vi "Main.vi"(10 "Parameters":variant, 11 "Process":refnum<class "Process.lvclass">) -> ()   [LabVIEW 2015, in "J1939 Addon Engine.lvlib"]
uses:
  J1939 Addon Engine.lvlib
  <vilib>/NI/NI VeriStand Inline Async API/_VS Inline Async API/Process/Process.lvclass
  Types/Process Parameters.ctl
  Shared/Types/XNET Settings.ctl
  Types/Incoming Single Point Configuration.ctl
  Types/Incoming Single Point Frame Pairs.ctl
  Shared/Types/Incoming Single Point Channel Pairs.ctl
  <vilib>/NI Veristand/Custom Device API/Data Reference.ctl
  Types/Outgoing Cyclic Configuration.ctl
  Types/Outgoing Cyclic Frame Pairs.ctl
  Shared/Types/XNET Frame Event Properties.ctl
  Shared/Types/Outgoing Cyclic Channel Pairs.ctl
  <vilib>/NI Veristand/Custom Device API/Block Data Reference.ctl
  Shared/Types/Monitor Settings.ctl
  Types/Simulated Settings.ctl
  Shared/Types/Compiled Simulated Settings.ctl
  Types/DTC FIFOs.ctl
  <vilib>/NI/NI VeriStand Inline Async API/_VS Inline Async API/Process/Process.lvclass/Process.ctl
  Shared/J1939 Multi Packet Frame/SubVIs/Convert Frame to NI-XNET CAN Frame.vi
  Shared/J1939 Multi Packet Frame/SubVIs/Listen for Claim.vi
  Shared/J1939 Multi Packet Frame/SubVIs/Address Claim Address.vi
  Shared/J1939 Utilities/Common Conversions.vi
  Shared/J1939 Utilities/SubVIs/Convert CAN Data (U8) to U32.vi
  Network Address Lookup Table.vi
  Shared/J1939 Multi Packet Frame/SubVIs/Cannont Claim Address.vi
  Shared/J1939 Utilities/SubVIs/Convert CAN Data (U32) to U8.vi
  Convert Signals to Frame by ID.vi
  Data Lookup Table Set Signals (Range).vi
  Data Lookup Table Get Signals (Range).vi
  <vilib>/NI/NI VeriStand Inline Async API/_VS Inline Async API/Process/Methods/Async.Processes.Report.vi
  Shared/J1939 Multi Packet Frame/Process Outgoing Messages.vi
  Shared/J1939 Multi Packet Frame/Check Outgoing TP Timeouts.vi
  Shared/J1939 Multi Packet Frame/SubVIs/Read Queued Processed Outgoing Messages.vi
  Shared/J1939 Multi Packet Frame/SubVIs/Read Queued Processed Incoming Messages.vi
  Conversion Lookup Table Get Conversion Parameter.vi
  Shared/J1939 Multi Packet Frame/SubVIs/RQST Look for Response.vi
  Shared/J1939 Multi Packet Frame/Check Incoming TP Timeouts.vi
  Shared/J1939 Multi Packet Frame/Process Incoming Messages.vi
  Shared/J1939 Multi Packet Frame/SubVIs/RQST Comm Lookup Table_Actions.vi
  Shared/J1939 Multi Packet Frame/SubVIs/RQST Wait on Response.vi
  Shared/J1939 Multi Packet Frame/SubVIs/RQST Wait on Multiple Requests.vi
  TCP Check Connection.vi
  Shared/STM/STM Get Connection Reference.vi
  Shared/STM/TCP/STM Get Connection Reference (TCP).vi
  <vilib>/Utility/error.llb/Clear Errors.vi
  Shared/J1939 Utilities/SubVIs/Convert CAN Arb ID to J1939 ID.vi
  Shared/J1939 Utilities/SubVIs/Convert J1939 ID to CAN Arb ID.vi
  <vilib>/NI/NI VeriStand Inline Async API/_VS Inline Async API/Error Handling Process/SubVIs/Error.ConvertArray.vi
  Shared/J1939 Multi Packet Frame/SubVIs/Read Queued Outgoing Messages.vi
  Shared/J1939 Multi Packet Frame/SubVIs/Process Outgoing Messages by Frame Type.vi
  Shared/J1939 Multi Packet Frame/J1939 Periodic Messages/Periodic Message Generator.vi
  Shared/J1939 Multi Packet Frame/SubVIs/Connection Mode Generation Queue Messages.vi
  Shared/J1939 Multi Packet Frame/SubVIs/RQST Lookup Table Act.vi
  Shared/J1939 Multi Packet Frame/J1939 Multi Packet Frames/BAM Buffer.vi
  Shared/J1939 Multi Packet Frame/SubVIs/TP Buffer Check Timeout on Connections.vi
  Shared/J1939 Multi Packet Frame/SubVIs/Buffer Connections List_Actions.vi
  Shared/J1939 Multi Packet Frame/J1939 Multi Packet Frames/Connnection Mode Buffer.vi
  Shared/J1939 Utilities/SubVIs/TP.Conn Abort.vi
  Shared/J1939 Utilities/Filter by Device Address.vi
  Shared/J1939 Multi Packet Frame/SubVIs/Process Incoming Messages by PDU F.vi
  Shared/J1939 Utilities/Common Messages.vi
  Shared/J1939 Utilities/SubVIs/Request.vi
  Shared/J1939 Utilities/Check Output Message Frame Type.vi
  Shared/J1939 Multi Packet Frame/J1939 Multi Packet Frames/BAM Generation.vi
  Shared/J1939 Multi Packet Frame/SubVIs/BAM Generation Connections List_Actions.vi
  Shared/J1939 Multi Packet Frame/SubVIs/BAM Generation Create New TP Connection.vi
  Shared/J1939 Multi Packet Frame/J1939 Multi Packet Frames/Connection Mode Generation.vi
  Shared/J1939 Multi Packet Frame/SubVIs/Connection Mode Generation Connections List_Actions.vi
  Shared/J1939 Multi Packet Frame/SubVIs/Connection Mode Generation Search for Connection (Local Message).vi
  Shared/J1939 Multi Packet Frame/SubVIs/Connection Mode Generation Create New TP Connection.vi
  Shared/J1939 Multi Packet Frame/SubVIs/Connection Mode Generation Get Next Messages.vi
  Shared/J1939 Utilities/Parse Message Type.vi
  Get Simulated Previously Active DTCs.vi
  Get Simulated Active DTCs.vi
  Shared/J1939 Utilities/SubVIs/Acknowledgement.vi
  Shared/J1939 Multi Packet Frame/SubVIs/TP Buffer Search for Connection (No PGN).vi
  Shared/J1939 Multi Packet Frame/SubVIs/TP Buffer Add New Data Packet to Connection.vi
  Shared/J1939 Multi Packet Frame/SubVIs/TP Buffer Convert Connection Info to CAN Frame.vi
  Shared/J1939 Multi Packet Frame/SubVIs/TP Buffer Create New TP Connection.vi
  Shared/J1939 Utilities/SubVIs/TP.CM EndofMsgACK.vi
  Shared/J1939 Utilities/SubVIs/TP.CM CTS.vi
  Shared/J1939 Multi Packet Frame/SubVIs/Connection Mode Generation Search for Connection (Remote Message).vi
  Shared/J1939 Multi Packet Frame/SubVIs/TP Buffer Search for Connection.vi
  Shared/J1939 Multi Packet Frame/SubVIs/Connection Mode Generation CTS Received.vi
  Shared/J1939 Utilities/SubVIs/TP.CM BAM.vi
  Shared/J1939 Utilities/SubVIs/TP.DT.vi
  Shared/J1939 Utilities/SubVIs/TP.CM RTS.vi
  Convert Data to DTC Frame.vi
  Shared/J1939 Utilities/SubVIs/Convert PGN + SA to J1939 ID.vi
  <vilib>/xnet/xnet.llb/XNET Convert.vi
  <vilib>/xnet/xnet.llb/XNET Convert (Signal to Frame Raw).vi
  Data Lookup Table.vi
  Conversion Lookup Table.vi
  Shared/J1939 Multi Packet Frame/SubVIs/Connection Mode Generation Connections List.vi
  Shared/J1939 Multi Packet Frame/SubVIs/BAM Generation Queue Messages.vi
  Shared/J1939 Multi Packet Frame/SubVIs/BAM Generation Connections List.vi
  Shared/J1939 Multi Packet Frame/SubVIs/BAM Generation Search for Connection (Local Message).vi
  <vilib>/xnet/xnet.llb/XNET Write.vi
  <vilib>/xnet/xnet.llb/XNET Write (Frame CAN).vi
  <vilib>/xnet/xnet.llb/XNET Convert (Frame CAN to Signal).vi
  Shared/J1939 Multi Packet Frame/SubVIs/RQST Lookup Table.vi
  Shared/J1939 Multi Packet Frame/SubVIs/BAM Buffer Connections List.vi
  Shared/J1939 Multi Packet Frame/SubVIs/Address Lookup Table.vi
  <vilib>/xnet/xnet.llb/XNET Read.vi
  <vilib>/xnet/xnet.llb/XNET Read (Frame CAN).vi
  Shared/STM/Clear Specific Error.vi
  Shared/STM/Connection Manager/TCP Connection Manager.vi
  <vilib>/NI Veristand/Custom Device Tools/Custom Device Utility Library/NI VeriStand - Print Debug String.vi
  Shared/STM/STM Read Meta Data.vi
  Shared/STM/TCP/STM Read Meta Data (TCP Ref).vi
  Shared/STM/STM Write Message.vi
  Shared/STM/TCP/STM Write Message (TCP).vi
  <vilib>/xnet/xnet.llb/XNET Read (State CAN Comm).vi
  <vilib>/Utility/error.llb/Error Cluster From Error Code.vi
  Shared/STM/STM Read Message.vi
  Shared/STM/TCP/STM Read Message (TCP).vi
  Shared/J1939 Utilities/SubVIs/Request Address.vi
  Shared/J1939 Addon Shared.lvlib
  <vilib>/NI VeriStand/Custom Device API/Custom Device API.lvlib
panel:
  out "error out":errorcluster
  # "CONTROL & MONITORING"
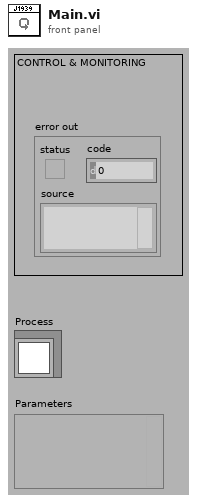
[diagram p1: front panel]
types:
  T1 = typedef "J1939 Addon Engine.lvlib/Process Parameters.ctl" = cluster{"J1939 XNET Settings":T2, "Incoming Single Point Configuraiton":T3, "Outgoing Cyclic Configuraiton":T7, "J1939 Monitor Settings":T12, "Simulated Addresses":T13[], "Simulated Addresses LUT":variant, "Name":string}
  T2 = typedef "J1939 Addon Shared.lvlib/XNET Settings.ctl" = cluster{"XNET Database":refnum<k21>, "XNET Cluster":refnum<k21>, "CAN Port":string, "Baud rate [Bd]":u32, "Termination":u32, "Incoming Rate":u32, "Outcoming Rate":u32, "Write Decimation":u32}
  T3 = typedef "J1939 Addon Engine.lvlib/Incoming Single Point Configuration.ctl" = cluster{"Incoming Single Point Frame":T4, "Channel Pairs":T5, "Read FIFO":refnum<k33>}
  T4 = typedef "J1939 Addon Engine.lvlib/Incoming Single Point Frame Pairs.ctl" = cluster{"ID":u32[], "Conversion":refnum<k21>[], "Channel Array Positions":cluster{"Offset":u32, "Length":u32}[], "Frame Length":u32[]}
  T5 = typedef "J1939 Addon Shared.lvlib/Incoming Single Point Channel Pairs.ctl" = cluster{"Chan Refs":T6[], "Previous Chan Values":dbl[]}
  T6 = typedef "Custom Device API.lvlib/Data Reference.ctl" = i32
  T7 = typedef "J1939 Addon Engine.lvlib/Outgoing Cyclic Configuration.ctl" = cluster{"Outgoing Cyclic Frame":T8, "Channel Pairs":T10, "Write FIFO":refnum<k33>}
  T8 = typedef "J1939 Addon Engine.lvlib/Outgoing Cyclic Frame Pairs.ctl" = cluster{"ID":u32[], "Conversion":refnum<k21>[], "Channel Array Positions":cluster{"Offset":u32, "Length":u32}[], "Frame Length":u32[], "Transmit Propreties":T9[]}
  T9 = typedef "J1939 Addon Shared.lvlib/XNET Frame Event Properties.ctl" = cluster{"Transmit trigger":enum16{"Channel value change"}, "Enable software cyclic trigger":bool, "Transmit Time":dbl}
  T10 = typedef "J1939 Addon Shared.lvlib/Outgoing Cyclic Channel Pairs.ctl" = cluster{"Block Data Refs":T11[], "Previous Chan Values":dbl[]}
  T11 = typedef "Custom Device API.lvlib/Block Data Reference.ctl" = cluster{"Data Reference":T6, "Offset":u64, "Length":u64}
  T12 = typedef "J1939 Addon Shared.lvlib/Monitor Settings.ctl" = cluster{"J1939 Network Address":u8, "Name":u64}
  T13 = typedef "J1939 Addon Engine.lvlib/Simulated Settings.ctl" = cluster{"Simulated Addresses":T14, "FIFOs":T15}
  T14 = typedef "J1939 Addon Shared.lvlib/Compiled Simulated Settings.ctl" = cluster{"J1939 XNET Settings":T12, "DM1 Data":T11[], "DM1 Data":dbl[], "DM1 Enable?":T11[], "DM1 Enable?":dbl[], "DM2 Data":T11[], "DM2 Data":dbl[], "DM2 Enable?":T11[], "DM2 Enable?":dbl[]}
  T15 = typedef "J1939 Addon Engine.lvlib/DTC FIFOs.ctl" = cluster{"DM1 Data":refnum<k33>, "DM1 Enable?":refnum<k33>, "DM2 Data":refnum<k33>, "DM2 Enable?":refnum<k33>, "DM1 Reset?":refnum<k33>, "DM2 Reset?":refnum<k33>}
  T16 = typedef "J1939 Addon Engine.lvlib/Configuration Cluster.ctl" = cluster{"Parameters":T1, "Name":string, "J1939 Cluster":T17, "References":T18, "Frame In":refnum<k21>, "Frame Out":refnum<k21>, "Incoming Timeout":u32, "Outgoing Timeout":u32, "Listener ID":refnum<k5>, "Process":refnum<class "Process.lvclass">, "Data Ref":T24, "Scale Ref":T25, "Incoming Direct Access":cluster{"Offset":u32, "Length":u32}, "Outgoing Direct Access":cluster{"Offset":u32, "Length":u32}, "TCP Mngr Ref":T26, "Name and Address":string, "Simulated Addresses":T13[], "Simulated Addresses LUT":variant}
  T17 = typedef "J1939 Addon Engine.lvlib/Setup Information Cluster.ctl" = cluster{"Processed Incoming":refnum<queue>, "Current Device Address":u8, "Processed Outgoing":refnum<queue>, "Process Outgoing":refnum<queue>, "Name":u64}
  T18 = typedef "J1939 Addon Engine.lvlib/TP List References.ctl" = cluster{"BAM Buffer":T19, "CM Buffer":T19, "CM Gen":T20, "BAM Gen":T21, "Address Claims":T22, "RQST":T23}
  T19 = typedef "J1939 Addon Engine.lvlib/BAM Buffer Connections List_Ref.ctl" = refnum<data-value>
  T20 = typedef "J1939 Addon Engine.lvlib/Connection Mode Generation Connection Ref.ctl" = refnum<data-value>
  T21 = typedef "J1939 Addon Engine.lvlib/BAM Generation Connections List_Ref.ctl" = refnum<data-value>
  T22 = typedef "J1939 Addon Engine.lvlib/Address Table Reference.ctl" = refnum<data-value>
  T23 = typedef "J1939 Addon Engine.lvlib/RQST Lookup Table Reference.ctl" = refnum<data-value>
  T24 = typedef "J1939 Addon Engine.lvlib/Data Lookup Table Reference.ctl" = refnum<data-value>
  T25 = typedef "J1939 Addon Engine.lvlib/Conversion Lookup Table Reference.ctl" = refnum<data-value>
  T26 = typedef "J1939 Addon Shared.lvlib/RQST Comm Lookup Table_Ref.ctl" = refnum<data-value>
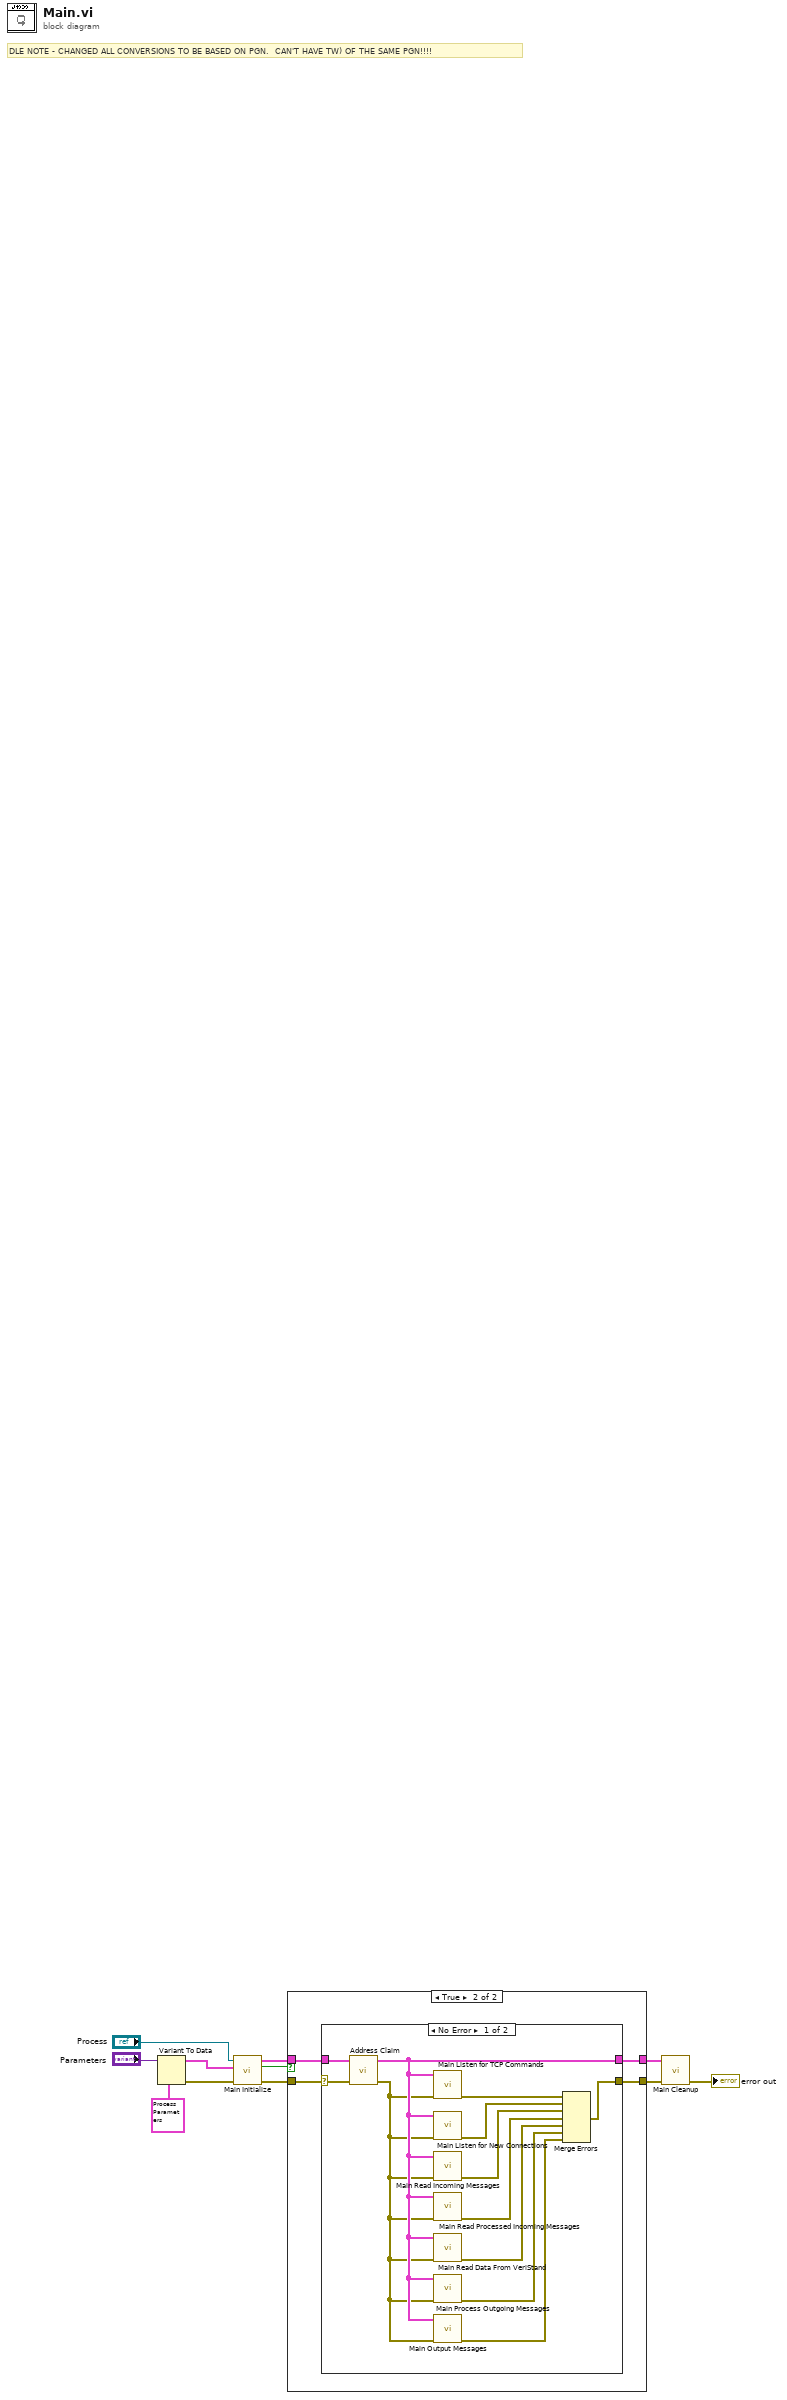
[diagram p0: block diagram]
diagram:
  # "DLE NOTE - CHANGED ALL CONVERSIONS TO BE BASED ON PGN.  CAN'T HAVE TW) OF THE SAME PGN!!!!"
  n1 = Variant To Data(type=T1 {"J1939 XNET Settings"={"XNET Database"="", "XNET Cluster"="", "CAN Port"="", "Baud rate [Bd]"=0, "Termination"=0, "Incoming Rate"=0, "Outcoming Rate"=1, "Write Decimation"=1}, "Incoming Single Point Configuraiton"={"Incoming Single Point Frame"={"ID"=[], "Conversion"=[], "Channel Array Positions"=[], "Frame Length"=[]}, "Channel Pairs"={"Chan Refs"=[], "Previous Chan Values"=[]}, "Read FIFO"=refnum}, "Outgoing Cyclic Configuraiton"={"Outgoing Cyclic Frame"={"ID"=[], "Conversion"=[], "Channel Array Positions"=[], "Frame Length"=[], "Transmit Propreties"=[]}, "Channel Pairs"={"Block Data Refs"=[], "Previous Chan Values"=[]}, "Write FIFO"=refnum}, "J1939 Monitor Settings"={"J1939 Network Address"=0, "Name"=0}, "Simulated Addresses"=[], "Simulated Addresses LUT"=variant, "Name"=""} ("Parameters"), Variant="Parameters") -> (data=w3:T1, error out=w2:errorcluster)  [unwired: 1 in]
  n2 = call "Main Initialize.vi"("error in (no error)"=w2, "Parameters in"=w3, "Process"="Process") -> ("error out"=w11:errorcluster, "Notification"=w8:bool, "J1939 Main Configuration"=w7:T16)  [unwired: 6 in]
  n3 = case shown="True" w8 {
    tunnel: w11 -> [w13 w16]
    tunnel: [w13 w17] -> w10
    tunnel: w7 -> [w12 w15]
    tunnel: [w12 w14] -> w6
    frame False {
    }
    frame True {
      n4 = case shown="No Error" w16 {
        selector: w16 -> [w23 w31]
        tunnel: [w29 w31] -> w17
        tunnel: w15 -> [w20 w30]
        tunnel: [w19 w30] -> w14
        frame No Error {
          n5 = call "Address Claim.vi"("error in (no error)"=w23, "J1939 Main Configuration"=w20) -> ("error out"=w18:errorcluster, "J1939 Main Configuration Out"=w19:T16)  [unwired: 8 in]
          n6 = call "Main Listen for TCP Commands.vi"("error in (no error)"=w18, "J1939 Main Configuration"=w19) -> ("error out"=w22:errorcluster)  [unwired: 9 in]
          n7 = call "Main Listen for New Connections.vi"("error in (no error)"=w18, "J1939 Main Configuration"=w19) -> ("error out"=w21:errorcluster)  [unwired: 9 in]
          n8 = call "Main Read Incoming Messages.vi"("error in (no error)"=w18, "J1939 Main Configuration"=w19) -> ("error out"=w28:errorcluster)  [unwired: 9 in]
          n9 = call "Main Read Processed Incoming Messages.vi"("error in (no error)"=w18, "J1939 Main Configuration"=w19) -> ("error out"=w27:errorcluster)  [unwired: 9 in]
          n10 = call "Main Read Data From VeriStand.vi"("error in (no error)"=w18, "J1939 Main Configuration"=w19) -> ("error out"=w26:errorcluster)  [unwired: 9 in]
          n11 = call "Main Process Outgoing Messages.vi"("error in (no error)"=w18, "J1939 Main Configuration"=w19) -> ("error out"=w25:errorcluster)  [unwired: 9 in]
          n12 = call "Main Output Messages.vi"("error in (no error)"=w18, "J1939 Main Configuration"=w19) -> ("error out"=w24:errorcluster)  [unwired: 9 in]
          n13 = Merge Errors(w22, w21, w28, w27, w26, w25, w24) -> (w29:errorcluster)
        }
        frame Error {
        }
      }
    }
  }
  n14 = call "Main Cleanup.vi"("error in (no error)"=w10, "J1939 Main Configuration"=w6) -> ("error out"=→"error out":errorcluster)  [unwired: 9 in]
